vi "GUI_about.vi"(4 "error in (no error)":errorcluster) -> (0 "error out":errorcluster)   [LabVIEW 2015]
panel:
  out "String":string="The Goodman spectrograph control system\nis written entirely in LabVIEW. It uses a thread/control reference architecture to coordinate the motions of 9 Silvermax smart motors, 2 stepper motors, and 2 piezo\nactuators. \n\nAuthor: \n\nJ Adam Crain\ncrain@physics.unc.edu\n"
  # "Goodman\nSpectrograph\nControl\nSystem"
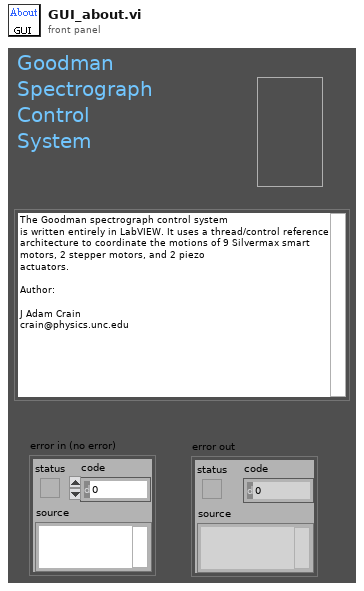
[diagram p1: front panel]
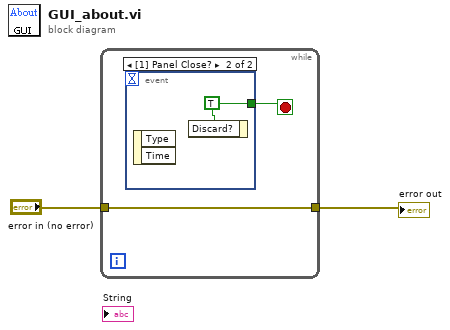
[diagram p0: block diagram]
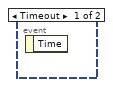
[diagram p2: hidden frame]
diagram:
  n1 = while {
    tunnel: [w4] -> w1
    tunnel: "error in (no error)" -> [w4]
    stop <- w3 stop-if-true
    n2 = event shown="[1] Panel Close?" {
      selector: _ -> [_ _]
      dyn-events: _ -> [_ _]
      timeout: _ -> [_ _]
      tunnel: [_ w5] -> w3
      event Timeout {
        n3 = event-data() -> ()  [unwired: 1 in, 1 out]
      }
      event Panel Close? {
        w5 = TRUE
        n4 = event-data() -> ()  [unwired: 1 in, 2 out]
        n5 = event-data("Discard?"=w5) -> ()  [unwired: 1 in, 1 out]
      }
    }
  }
  "error out" <- w1
